vi "Actor Core.vi"(8 "error in":errorcluster, 11 "WS Test Server in":refnum<class "WS Server.lvclass">) -> (0 "error out":errorcluster, 3 "Actor out":refnum<class "Actor.lvclass">)   [LabVIEW 2021, in "Echo Broadcast with External Client.lvlib" / "WS Server.lvclass"]
doc: "(<B>Filename</B>: Actor Framework.lvlib:Actor.lvclass:Actor Core.vi)\n\nReceives messages to the actor, reacts to them, and initiates any error handling that may shut the actor down.\n\nDescendant classes may override this VI to append parallel tasks for the actor to complete while it handles messages. Overrides use the Call Parent Method node."
uses:
  WS Server.lvclass
  <vilib>/ActorFramework/Actor/Actor.lvclass
  C:/Program Files/National Instruments/LabVIEW 2021/vi.lib/ActorFramework/Actor/Actor.lvclass
  WebSocket Actor/WebSocket Server/typedefs/Listener Settings.ctl
  <vilib>/ActorFramework/Message Enqueuer/Message Enqueuer.lvclass
  <vilib>/ActorFramework/Actor/Actor.lvclass/Actor.ctl
  <vilib>/ActorFramework/Message Enqueuer/Message Enqueuer.lvclass/Message Enqueuer.ctl
  WS Server.lvclass/WS Server.ctl
  WS Server Messages/WebSocket Server Enqueuer Msg/WebSocket Server Enqueuer Msg.lvclass
  C:/Projects/WebSocket-Actor/WebSocket Actor/Abstract Messages/WebSocket Server-Service Enqueuer Msg/WebSocket Server-Service Enqueuer Msg.lvclass
  WS Server Messages/Server Connection Handler Msg/Server Connection Handler Msg.lvclass
  C:/Projects/WebSocket-Actor/WebSocket Actor/Abstract Messages/WebSocket Connection Handler Msg/WebSocket Connection Handler Msg.lvclass
  <vilib>/ActorFramework/Message Enqueuer/Init from Existing Queue.vi
  <vilib>/ActorFramework/Message Enqueuer/Enqueue.vi
  <vilib>/ActorFramework/Stop Msg/Stop Msg.lvclass
  C:/Program Files/National Instruments/LabVIEW 2021/vi.lib/ActorFramework/Message/Message.lvclass
  <vilib>/Utility/LVClass/Get LV Class Name.vi
  <resource>/AFDebug/Generate Trace for Message.vi
  <vilib>/ActorFramework/Message Priority Queue/Priority Enqueue.vi
  WebSocket Actor/WebSocket Server Manager Messages/Launch Server Msg/Launch Server Msg.lvclass
  WebSocket Actor/WebSocket Server Manager Messages/Stop Server Msg/Stop Server Msg.lvclass
  WebSocket Actor/WebSocket Server/WebSocket Server.lvclass
  WebSocket Actor/WebSocket Server Messages/Add Service Msg/Add Service Msg.lvclass
panel:
  in  "Service":string="/echo"
  in  "Add Service":bool
  in  "Listener Settings":T1={"resolve remote address (T)"=TRUE, "timeout ms (-1)"=-1, "net address"=0, "port"=6163}
  in  "Handshake timeout (5000 ms)":i32=5000
  in  "Stop Server":bool
  in  "Launch Server":bool
  in  "Exit":bool
  out "Launch/Stop Error":errorcluster
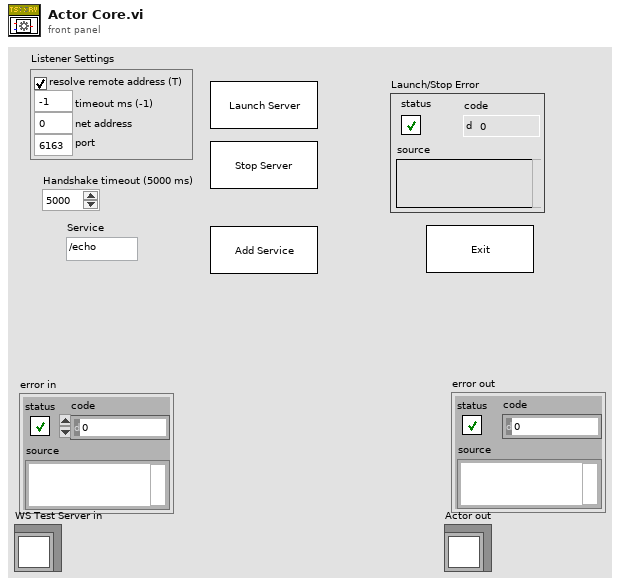
[diagram p1: front panel]
types:
  T1 = typedef "WebSocket Actors.lvlib/WebSocket Server.lvclass/Listener Settings.ctl" = cluster{"resolve remote address (T)":bool, "timeout ms (-1)":i32, "net address":u32, "port":u16}
  T2 = enum8{"Enabled", "Disabled", "Disabled and Grayed Out"}
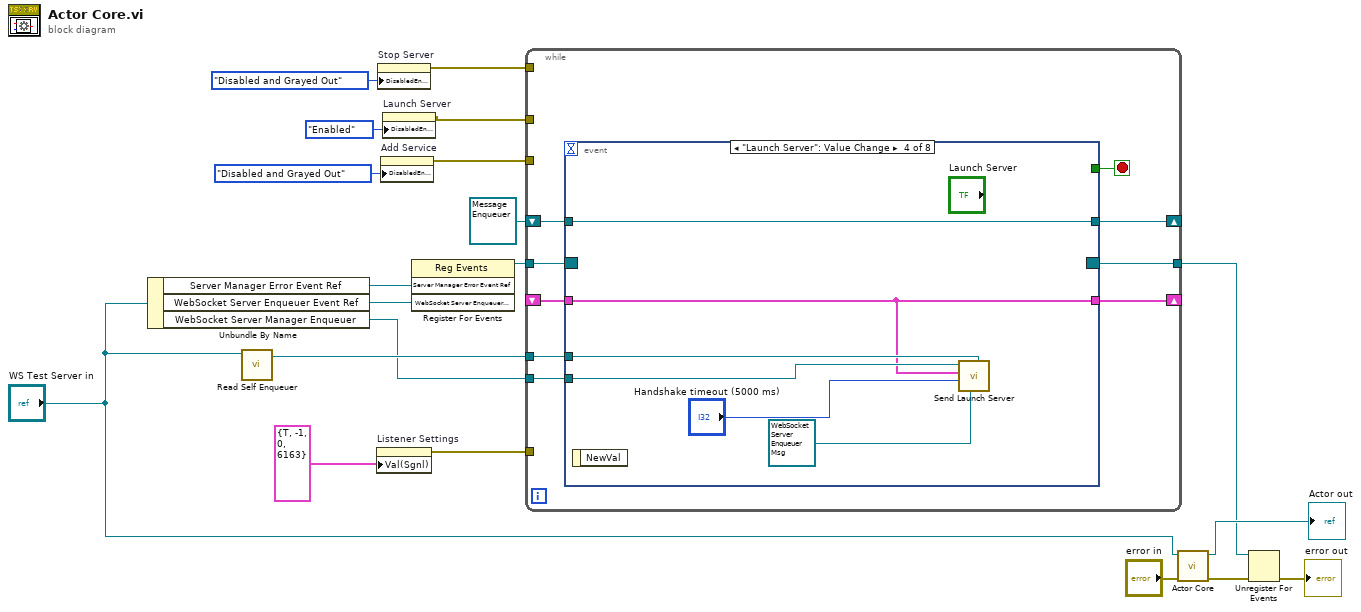
[diagram p0: block diagram]
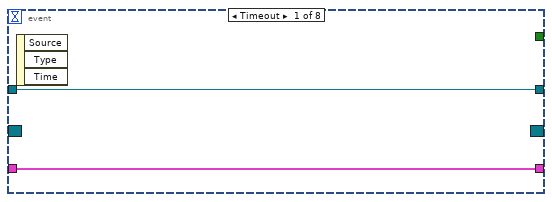
[diagram p2: hidden frame]
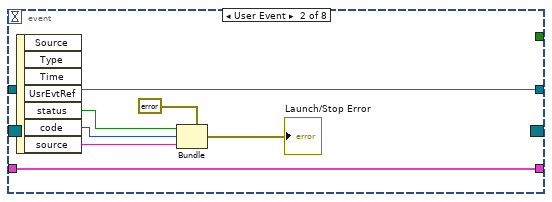
[diagram p3: hidden frame]
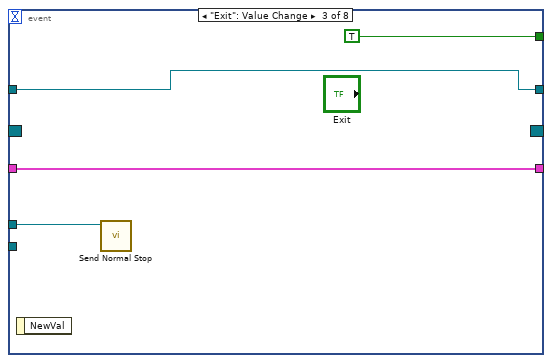
[diagram p4: hidden frame]
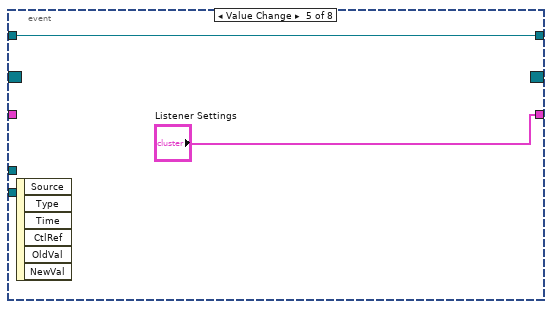
[diagram p5: hidden frame]
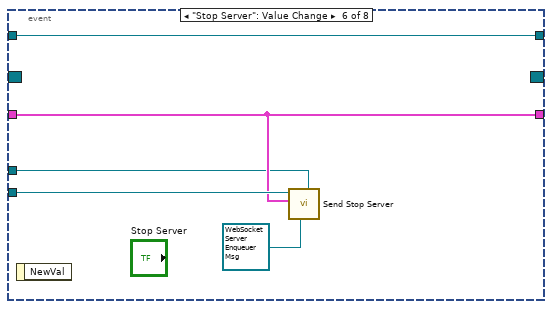
[diagram p6: hidden frame]
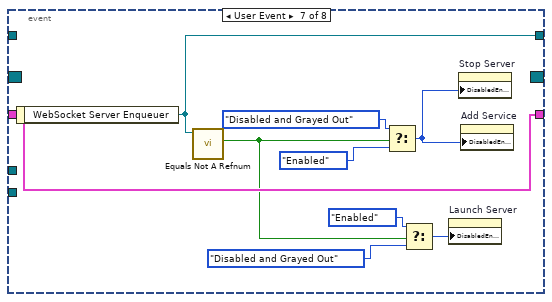
[diagram p7: hidden frame]
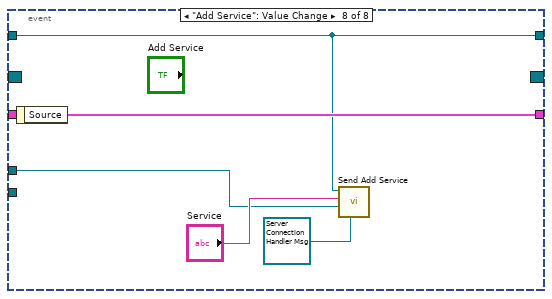
[diagram p8: hidden frame]
diagram:
  n1 = Unbundle By Name("WS Test Server in") -> ("Server Manager Error Event Ref"=w18:refnum<user-event>, "WebSocket Server Enqueuer Event Ref"=w9:refnum<user-event>, "WebSocket Server Manager Enqueuer"=w8:refnum<class "Message Enqueuer.lvclass">)
  n2 = call <vilib>:"Read Self Enqueuer.vi"("Actor"="WS Test Server in") -> ("Self Enqueuer"=w14:refnum<class "Message Enqueuer.lvclass">)  [unwired: 10 in]
  n3 = property on="Listener Settings" class="Clust (strict)"("Val(Sgnl)"=T1 {"resolve remote address (T)"=TRUE, "timeout ms (-1)"=-1, "net address"=0, "port"=6163} ("Listener Settings")) -> (error out=w10:errorcluster)  [unwired: 2 in, 1 out]
  n4 = property on="Stop Server" class="Bool"("DisabledEnum"=T2."Disabled and Grayed Out" ("Disabled")) -> (error out=w1:errorcluster)  [unwired: 2 in, 1 out]
  n5 = property on="Add Service" class="Bool"("DisabledEnum"=T2."Disabled and Grayed Out" ("Disabled")) -> (error out=w5:errorcluster)  [unwired: 2 in, 1 out]
  n6 = property on="Launch Server" class="Bool"("DisabledEnum"=T2."Enabled" ("Disabled")) -> (error out=w3:errorcluster)  [unwired: 2 in, 1 out]
  n7 = register-events(w18, w9) -> (reference out=w17:refnum<event-registration>)  [unwired: 2 in, 1 out]
  n8 = while {
    tunnel: w17 -> [w29]
    tunnel: [w28] -> w15
    tunnel: w8 -> [w26]
    tunnel: w14 -> [w25]
    shift-right: [w24] -> _
    shift-left: _ -> [w23]
    tunnel: w10 -> [_]
    shift-right: [w22] -> _
    shift-left: refnum<class "Message Enqueuer.lvclass"> refnum ("WebSocket Server Enqueuer") -> [w21]
    tunnel: w5 -> [_]
    tunnel: w3 -> [_]
    tunnel: w1 -> [_]
    stop <- w27 stop-if-true
    n9 = event shown="[3] \"Launch Server\": Value Change" {
      selector: w29 -> [_ _ _ _ _ _ _ _]
      dyn-events: [_ _ _ _ _ _ _ _] -> w28
      timeout: _ -> [_ _ _ _ _ _ _ _]
      tunnel: [_ _ TRUE _ _ _ _ _] -> w27
      tunnel: w26 -> [_ _ _ w47 _ w55 _ _]
      tunnel: w25 -> [_ _ w41 w46 _ w52 _ w66]
      tunnel: [w31 w33 w40 w44 "Listener Settings" w54 w61 w69] -> w24
      tunnel: w23 -> [w31 w33 w40 w44 _ w54 w61 w69]
      tunnel: [w30 w32 w39 w43 w49 w51 w64 w68] -> w22
      tunnel: w21 -> [w30 w32 w39 w43 w49 w51 _ w68]
      event Timeout {
        n10 = event-data() -> ()  [unwired: 1 in, 3 out]
      }
      event User Event {
        n11 = event-data() -> ("status"=w37:bool, "code"=w36:i32, "source"=w35:string)  [unwired: 1 in, 4 out]
        n12 = Bundle(cluster=errorcluster {"status"=FALSE, "code"=0, "source"=""} ("error out 2"), "status"=w37, "code"=w36, "source"=w35) -> (→"Launch/Stop Error":errorcluster)
      }
      event "Exit": Value Change {
        n13 = event-data() -> ()  [unwired: 1 in, 1 out]
        n14 = call <vilib>:"Send Normal Stop.vi"("Message Enqueuer"=w41) -> ()  [unwired: 10 in, 1 out]
      }
      event "Launch Server": Value Change {
        n15 = event-data() -> ()  [unwired: 1 in, 1 out]
        n16 = call "Send Launch Server.vi"("Subscriber Enqueuer"=w46, "Receive Server Enqueuer Handler"=refnum<class "WebSocket Server Enqueuer Msg.lvclass"> refnum ("Echo Broadcast Test With Server Manager.lvlib:WebSocket Server Enqueuer Msg.lvclass"), "Handshake timeout (5000 ms)"="Handshake timeout (5000 ms)", "Listener Settings"=w44, "Message Enqueuer in"=w47) -> ()  [unwired: 5 in, 2 out]
      }
      event Value Change {
        n17 = event-data() -> ()  [unwired: 1 in, 6 out]
      }
      event "Stop Server": Value Change {
        n18 = event-data() -> ()  [unwired: 1 in, 1 out]
        n19 = call "Send Stop Server.vi"("Subscriber Enqueuer"=w52, "Receive Server Enqueuer Handler"=refnum<class "WebSocket Server Enqueuer Msg.lvclass"> refnum ("Echo Broadcast Test With Server Manager.lvlib:WebSocket Server Enqueuer Msg.lvclass"), "Listener Settings"=w54, "Message Enqueuer in"=w55) -> ()  [unwired: 6 in, 2 out]
      }
      event User Event {
        n20 = event-data() -> ("WebSocket Server Enqueuer"=w64:refnum<class "Message Enqueuer.lvclass">)  [unwired: 1 in]
        n21 = call <vilib>:"Equals Not A Refnum.vi"("Message Enqueuer"=w64) -> ("Not a refnum?"=w56:bool)  [unwired: 10 in]
        n22 = Select(t=T2."Disabled and Grayed Out" ("Disabled"), s=w56, f=T2."Enabled" ("Disabled")) -> (s? t:f=w60:T2)
        n23 = Select(t=T2."Enabled" ("Disabled"), s=w56, f=T2."Disabled and Grayed Out" ("Disabled")) -> (s? t:f=w57:T2)
        n24 = property on="Launch Server" class="Bool"("DisabledEnum"=w57) -> ()  [unwired: 2 in, 2 out]
        n25 = property on="Stop Server" class="Bool"("DisabledEnum"=w60) -> ()  [unwired: 2 in, 2 out]
        n26 = property on="Add Service" class="Bool"("DisabledEnum"=w60) -> ()  [unwired: 2 in, 2 out]
      }
      event "Add Service": Value Change {
        n27 = event-data() -> ()  [unwired: 1 in, 1 out]
        n28 = call "Send Add Service.vi"("WebSocket Data Handler"=refnum<class "Server Connection Handler Msg.lvclass"> refnum ("Echo Broadcast with External Client.lvlib:Server Connection Handler Msg.lvclass"), "Subscriber Enqueuer"=w66, "Service Name"="Service", "Message Enqueuer in"=w68) -> ()  [unwired: 6 in, 2 out]
      }
    }
  }
  n29 = call-parent "Actor Core.vi"("error in"="error in", "Actor in"="WS Test Server in") -> ("error out"=w13:errorcluster, "Actor out"=→"Actor out":refnum<class "Actor.lvclass">)  [unwired: 8 in]
  n30 = Unregister For Events(event registration refnum=w15, error in=w13) -> (error out=→"error out":errorcluster)
